vi "Xml_Save_Spectrum.vi"(8 "error in (no error)":errorcluster, 10 "Refnum Cluster\nEXPERT":refnum<vi>, 11 "Refnum Cluster\nSPECTRUM":refnum<vi>) -> (0 "error out":errorcluster, 3 "XML String Out":string)   [LabVIEW 2024]
uses:
  controls/EXPERT_Inputs.ctl
  controls/XML_Inputs.ctl
  controls/SOFTWARE_Inputs.ctl
  controls/HSDIO_6541_Inputs.ctl
  <instrlib>/niHSDIO/niHSDIO.llb/niHSDIO_ctl Trigger Source Values (Ring).ctl
  controls/AWG_5421_Inputs.ctl
  <instrlib>/niFgen/niFgen.llb/niFgen_ctl Trigger Source Values (Ring).ctl
  controls/DIGIT_5122_Inputs.ctl
  <instrlib>/niScope/Controls/niScope trigger source.ctl
  controls/AO_6711_Inputs.ctl
  controls/AO_6738_Inputs.ctl
  controls/SPECTRUM.ctl
  <vilib>/NI/GXML/GXML.lvlib
panel:
  in  "EXPERT Inputs":T1={"XML Inputs"={"Version Tag Name"="XML_Version", "Version String"="1.0"}, "SOFTWARE Inputs"={"Application Directory"=path "D:/S.O.F.T.S/LABVIEW/PIL", "Software Version"="1.0.0", "Data Path"=path "D:/PIRENEA/DATA", "XML Path"=path "D:/PIRENEA/DATA", "XML File Filter"="*.xml", "XML Saved Path"=path "D:/PIRENEA/DATA/SAVED", "Excit Scripts Path"=path "D:/PIRENEA/EXCIT_SCRIPTS", "Excit Scripts File Filter"="*.txt", "Excit Waveforms Path"=path "D:/PIRENEA/EXCIT_WFMS", "Excit Waveforms File Filter"="*.bin", "Timing Scripts Path"=path "D:/PIRENEA/TIMING_SCRIPTS", "Timing Scripts File Filter"="*.txt", "Timing Waveforms Path"=path "D:/PIRENEA/TIMING_WFMS", "Timing Waveforms File Filter"="*.bin", "Trapping Waveforms Path"=path "D:/PIRENEA/TRAPPING_WFMS", "Trapping Waveforms File Filter"="*.bin"}, "HSDIO 6541 Inputs"={"Resource Name"="HSDIO_6541", "Clock Rate"=1000000.0, "Trigger Source"="PFI0"}, "AWG 5421 Inputs"={"Resource Name"="AWG_5421", "Sample Rate"=10000000.0, "Trigger Type"=2, "Trigger Source"="PFI0", "Waveform Gain"=0.31, "Digital Filter ON"=TRUE}, "DIGIT 5122 Inputs"={"Sample Rate"=10000.0, "Resource Name"="DIGIT_5122", "Channel Name"="0", "Trigger Source"="VAL_EXTERNAL", "Vertical Range"=10.0, "Trigger Level"=3.0}, "AO 6711 Inputs"={"Physical Channels"="AO_6711/ao0:3", "Min Voltage"=-10.0, "Max Voltage"=10.0, "Trigger Source"="/AO_6711/PFI3", "Counter"="AO_6711/ctr0"}, "AO 6738 Inputs"={"Physical Channels"="AO_6738/ao0:3", "Min Voltage"=-10.0, "Max Voltage"=10.0, "Trigger Source"="/AO_6738/PFI2", "Counter"="AO_6738/ctr0"}} {"AO 6738 Inputs"."Max Voltage" min=-10.0 max=10.0; "AO 6738 Inputs"."Min Voltage" min=-10.0 max=10.0; "AWG 5421 Inputs"."Sample Rate" format="%.2p"; "AWG 5421 Inputs"."Trigger Type" items=["None", "Software Edge", "Digital Edge", "Digital Level"]; "AO 6711 Inputs"."Max Voltage" min=-10.0 max=10.0; "AO 6711 Inputs"."Min Voltage" min=-10.0 max=10.0; "HSDIO 6541 Inputs"."Clock Rate" format="%.2p"; "DIGIT 5122 Inputs"."Trigger Level" format="%.2f"; "DIGIT 5122 Inputs"."Vertical Range" format="%.2f"; "DIGIT 5122 Inputs"."Sample Rate" step=65535.0 format="%#_3p"}
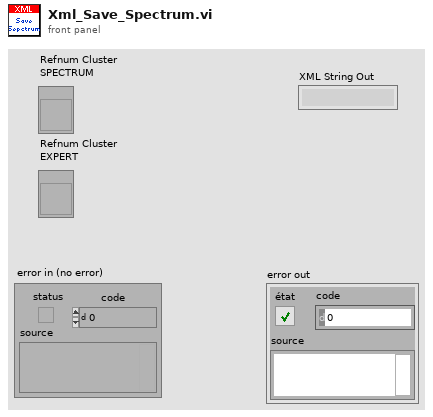
[diagram p1: front panel]
types:
  T1 = typedef "EXPERT_Inputs.ctl" = cluster{"XML Inputs":T2, "SOFTWARE Inputs":T3, "HSDIO 6541 Inputs":T4, "AWG 5421 Inputs":T6, "DIGIT 5122 Inputs":T8, "AO 6711 Inputs":T10, "AO 6738 Inputs":T11}
  T2 = typedef "XML_Inputs.ctl" = cluster{"Version Tag Name":string, "Version String":string}
  T3 = typedef "SOFTWARE_Inputs.ctl" = cluster{"Application Directory":path, "Software Version":string, "Data Path":path, "XML Path":path, "XML File Filter":string, "XML Saved Path":path, "Excit Scripts Path":path, "Excit Scripts File Filter":string, "Excit Waveforms Path":path, "Excit Waveforms File Filter":string, "Timing Scripts Path":path, "Timing Scripts File Filter":string, "Timing Waveforms Path":path, "Timing Waveforms File Filter":string, "Trapping Waveforms Path":path, "Trapping Waveforms File Filter":string}
  T4 = typedef "HSDIO_6541_Inputs.ctl" = cluster{"Resource Name":refnum<k15>, "Clock Rate":dbl, "Trigger Source":T5}
  T5 = typedef "niHSDIO_ctl Trigger Source Values (Ring).ctl" = string
  T6 = typedef "AWG_5421_Inputs.ctl" = cluster{"Resource Name":refnum<k15>, "Sample Rate":dbl, "Trigger Type":u16, "Trigger Source":T7, "Waveform Gain":dbl, "Digital Filter ON":bool}
  T7 = typedef "niFgen_ctl Trigger Source Values (Ring).ctl" = string
  T8 = typedef "DIGIT_5122_Inputs.ctl" = cluster{"Sample Rate":dbl, "Resource Name":refnum<k15>, "Channel Name":string, "Trigger Source":T9, "Vertical Range":dbl, "Trigger Level":dbl}
  T9 = typedef "niScope trigger source.ctl" = string
  T10 = typedef "AO_6711_Inputs.ctl" = cluster{"Physical Channels":tag, "Min Voltage":dbl, "Max Voltage":dbl, "Trigger Source":tag, "Counter":tag}
  T11 = typedef "AO_6738_Inputs.ctl" = cluster{"Physical Channels":tag, "Min Voltage":dbl, "Max Voltage":dbl, "Trigger Source":tag, "Counter":tag}
  T12 = typedef "SPECTRUM.ctl" = cluster{"Day Path":path, "Spectrum Name":string, "Accumulated":bool, "Stored in Database":bool, "From a Set of":i16, "Quality Flag":string}
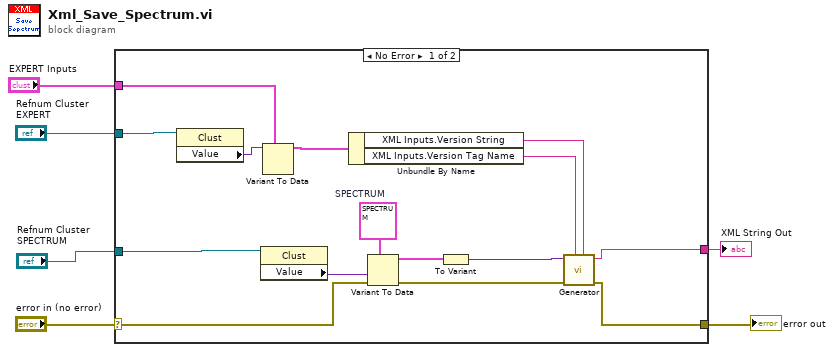
[diagram p0: block diagram]
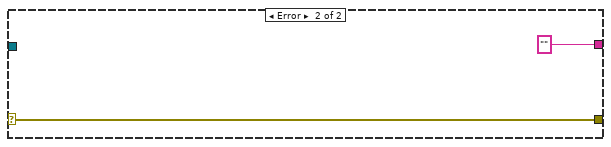
[diagram p2: hidden frame]
diagram:
  n1 = case shown="No Error" "error in (no error)" {
    selector: "error in (no error)" -> [w7 w23]
    tunnel: [w17 w23] -> w5
    tunnel: [w20 "" ("XML String Out")] -> w4
    tunnel: "Refnum Cluster\nSPECTRUM" -> [w13 _]
    tunnel: "Refnum Cluster\nEXPERT" -> [w21 _]
    tunnel: "EXPERT Inputs" -> [w14 _]
    frame No Error {
      w11 = T12 {"Day Path"=path "D:/PIRENEA/DATA/2016/data_2016_01_01", "Spectrum Name"="2016_01_01_000.A00", "Accumulated"=FALSE, "Stored in Database"=FALSE, "From a Set of"=1, "Quality Flag"="Optimal"}  # SPECTRUM
      n2 = property class="Clust"(reference=w21) -> ("Value"=w19:variant)  [unwired: 1 in, 2 out]
      n3 = property class="Clust"(reference=w13) -> ("Value"=w12:variant)  [unwired: 1 in, 2 out]
      n4 = Variant To Data(type=w14, Variant=w19) -> (data=w18:T1)  [unwired: 1 in, 1 out]
      n5 = Unbundle By Name(w18) -> ("XML Inputs.Version String"=w15:string, "XML Inputs.Version Tag Name"=w16:string)
      n6 = Variant To Data(error in=w7, type=w11, Variant=w12) -> (data=w10:T12, error out=w8:errorcluster)
      n7 = To Variant(anything=w10) -> (Variant=w9:variant)
      n8 = call <vilib>:"Generator.vi"("Version String"=w15, "Version Tag Name"=w16, "error in"=w8, "Variant"=w9) -> ("error out"=w17:errorcluster, "XML String Out"=w20:string)  [unwired: 6 in]
    }
    frame Error {
    }
  }
  "error out" <- w5
  "XML String Out" <- w4
